vi "Ticks To Radians.vi"() -> ()   [LabVIEW 2018]
panel:
  in  "Ticks/Rev":i32=4096
  out "Radians":dbl
  in  "Ticks":dbl
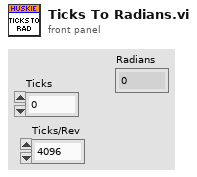
[diagram p1: front panel]
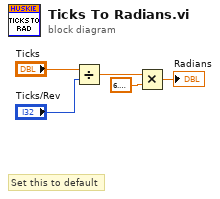
[diagram p0: block diagram]
diagram:
  # "Set this to default"
  n1 = Divide(x="Ticks", y="Ticks/Rev") -> (x/y=w4:dbl)
  n2 = Multiply(x=w4, y=6.283185307179586) -> (x*y=→"Radians":dbl)
